vi "Get Device Configuration.vi"(11 "SOL MS in":refnum<class "PL SOL Instruments MS.lvclass">) -> (2 "configuration":T1, 3 "SOL MS out":refnum<class "PL SOL Instruments MS.lvclass">)   [LabVIEW 2015, in "PL SOL Instruments MS.lvclass"]
doc: "Returns current device configuration."
uses:
  PL SOL Instruments MS.lvclass
  PL SOL Instruments MS.lvclass/PL SOL Instruments MS.ctl
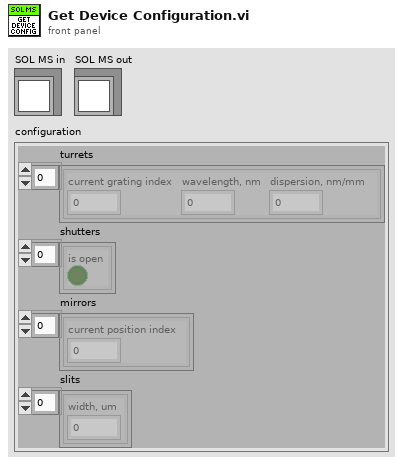
[diagram p1: front panel]
types:
  T1 = cluster{"turrets":cluster{"current grating index":u8, "wavelength, nm":dbl, "dispersion, nm/mm":dbl}[], "shutters":cluster{"is open":bool}[], "mirrors":cluster{"current position index":u8}[], "slits":cluster{"width, um":dbl}[]}
  T2 = cluster{"name":string, "step timeout, ms":u32, "reset timeout, ms":u32, "gratings":cluster{"name":string, "step timeout, ms":u32, "reset timeout, ms":u32, "turret position":i32, "reset position":i32, "max position":i32, "backlash distance":i32, "step size, rad":dbl, "groove density, g/mm":dbl, "theta2, rad":dbl, "blaze wavelength, nm":dbl, "focal length, cm":dbl, "manual change":bool, "manual change position":i32}[], "current grating":cluster{"index":u8, "position":i32}}[]
  T3 = cluster{"name":string, "step timeout, ms":u32, "reset timeout, ms":u32, "positions":cluster{"name":string, "position":i32}[], "current position index":u8}[]
  T4 = cluster{"name":string, "step timeout, ms":u32, "reset position":i32, "max position":i32, "backlash distance":i32, "step size, um":dbl, "current position":i32}[]
  T5 = cluster{"current grating index":u8, "wavelength, nm":dbl, "dispersion, nm/mm":dbl}[]
  T6 = cluster{"current grating index":u8, "wavelength, nm":dbl, "dispersion, nm/mm":dbl}
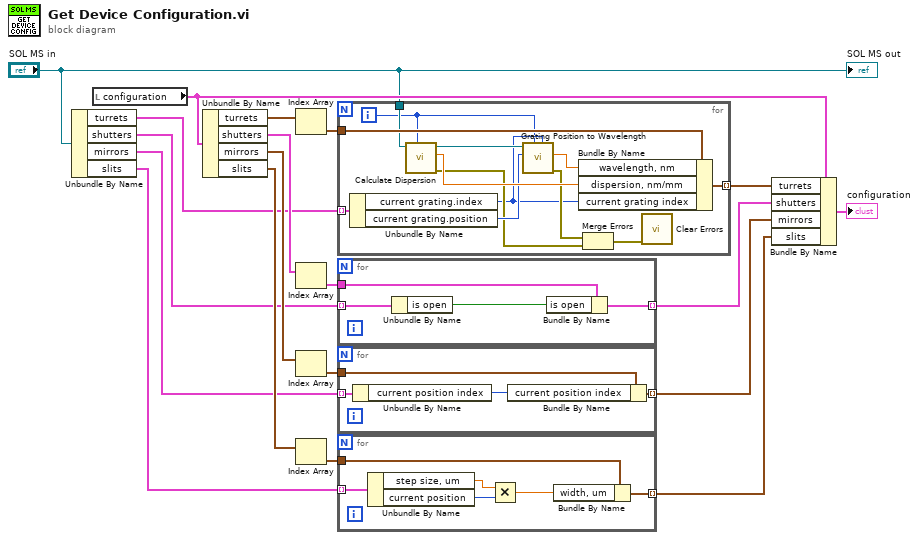
[diagram p0: block diagram]
diagram:
  n1 = Unbundle By Name("SOL MS in") -> ("turrets"=w15:T2, "shutters"=w11:cluster{"name":string, "is open":bool}[], "mirrors"=w8:T3, "slits"=w4:T4)
  n2 = local read "configuration"() -> (w3:T1)
  n3 = Unbundle By Name(w3) -> ("turrets"=w19:T5, "shutters"=w18:cluster{"is open":bool}[], "mirrors"=w17:cluster{"current position index":u8}[], "slits"=w16:cluster{"width, um":dbl}[])
  n4 = Index Array(array=w19) -> (element=w13:T6)  [unwired: 1 in]
  n5 = Index Array(array=w18) -> (element=w12:cluster{"is open":bool})  [unwired: 1 in]
  n6 = Index Array(array=w17) -> (element=w9:cluster{"current position index":u8})  [unwired: 1 in]
  n7 = Index Array(array=w16) -> (element=w5:cluster{"width, um":dbl})  [unwired: 1 in]
  n8 = for {
    tunnel: w15 -> [w32] mode=indexing
    tunnel: [w31] -> w14 mode=indexing
    tunnel: w13 -> [w30]
    tunnel: "SOL MS in" -> [w29]
    i -> [w20]
    n9 = Unbundle By Name(w32) -> ("current grating.index"=w21:u8, "current grating.position"=w25:i32)
    n10 = call "Calculate Dispersion.vi"("turret index (0)"=w20, "SOL MS in"=w29) -> ("error out"=w23:errorcluster, "dispersion, nm/mm"=w28:dbl, "SOL MS out"=w27:refnum<class "PL SOL Instruments MS.lvclass">)  [unwired: 7 in]
    n11 = call "Grating Position to Wavelength.vi"("grating index (0)"=w21, "turret index (0)"=w20, "grating position"=w25, "SOL MS in"=w27) -> ("error out"=w24:errorcluster, "wavelength, nm"=w26:dbl)  [unwired: 5 in, 1 out]
    n12 = Bundle By Name(cluster=w30, "wavelength, nm"=w26, "dispersion, nm/mm"=w28, "current grating index"=w21) -> (w31:T6)
    n13 = Merge Errors(w24, w23) -> (w22:errorcluster)
    n14 = call <vilib>:"Clear Errors.vi"("error in (no error)"=w22) -> ()  [unwired: 5 in, 2 out]
  }
  n15 = for {
    tunnel: w11 -> [w36] mode=indexing
    tunnel: [w34] -> w10 mode=indexing
    tunnel: w12 -> [w33]
    n16 = Unbundle By Name(w36) -> ("is open"=w35:bool)
    n17 = Bundle By Name(cluster=w33, "is open"=w35) -> (w34:cluster{"is open":bool})
  }
  n18 = for {
    tunnel: w8 -> [w40] mode=indexing
    tunnel: [w38] -> w7 mode=indexing
    tunnel: w9 -> [w37]
    n19 = Unbundle By Name(w40) -> ("current position index"=w39:u8)
    n20 = Bundle By Name(cluster=w37, "current position index"=w39) -> (w38:cluster{"current position index":u8})
  }
  n21 = for {
    tunnel: w4 -> [w46] mode=indexing
    tunnel: [w45] -> w6 mode=indexing
    tunnel: w5 -> [w44]
    n22 = Unbundle By Name(w46) -> ("step size, um"=w41:dbl, "current position"=w43:i32)
    n23 = Multiply(x=w41, y=w43) -> (x*y=w42:dbl)
    n24 = Bundle By Name(cluster=w44, "width, um"=w42) -> (w45:cluster{"width, um":dbl})
  }
  n25 = Bundle By Name(cluster=w3, "turrets"=w14, "shutters"=w10, "mirrors"=w7, "slits"=w6) -> (→"configuration":T1)
  "SOL MS out" <- "SOL MS in"
